vi "sub_slope2angle.vi"(11 "slope":dbl) -> (3 "angle deg":dbl)   [LabVIEW 2018]
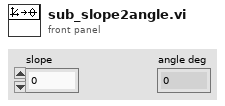
[diagram p1: front panel]
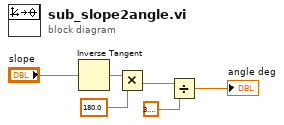
[diagram p0: block diagram]
diagram:
  n1 = Inverse Tangent(1:"slope") -> (0:w6:dbl)
  n2 = Multiply(x=w6, y=180.0) -> (x*y=w3:dbl)
  n3 = Divide(x=w3, y=3.141592653589793) -> (x/y=→"angle deg":dbl)
